vi "soft heap limit.vi"(8 "error in (no error)":errorcluster, 11 "N":i32) -> (0 "error out":errorcluster)   [LabVIEW 2020, in "sqlite3.lvlib"]
uses:
  sqlite3.lvlib
  errstr.vi
  bin/sqlite3_64.dll
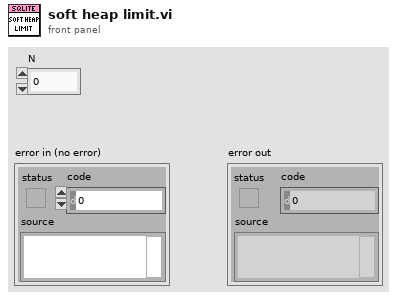
[diagram p1: front panel]
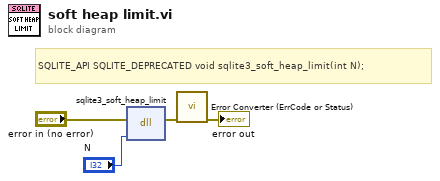
[diagram p0: block diagram]
diagram:
  # "SQLITE_API SQLITE_DEPRECATED void sqlite3_soft_heap_limit(int N);"
  n1 = dll-call lib="C:/Users/Fred.Guo/Desktop/Database-configuration/externals/sqlite3/Source/bin/sqlite3_*.*" fn="sqlite3_soft_heap_limit"(error in="error in (no error)", "N"="N") -> (error out=w2:errorcluster)  [unwired: 4 in, 1 out]
  n2 = call "Error Converter (ErrCode or Status).vi"("error in (no error)"=w2) -> ("error out"=→"error out":errorcluster)  [unwired: 10 in]
